vi "api_mqttSubscribe.vi"(0 "mqtt in":refnum<class "mqtt.lvclass">, 5 "subscriptionInfo":T1[](array[typedef])=[{"Topic"="a/b", "QoS"=enum."At least once"}], 9 "messageID":u16, 11 "error in (no error)":errorcluster) -> (4 "mqtt out":refnum<class "mqtt.lvclass">, 6 "success":bool, 15 "error out":errorcluster)   [LabVIEW 2020, in "mqtt.lvclass"]
uses:
  mqtt.lvclass
  mqttTypedef/mqttSubscribeCluster.ctl
  mqttTypedef/mqttQOSlevel.ctl
  mqttCmd/mqttCmdSubscribe/SubscribeMqttMsg.lvclass
  C:/Projects/Libraries/Gore SM 2020/mqtt-LabVIEW/src/class/mqtt/mqttCmd/BaseMqttMsg.lvclass
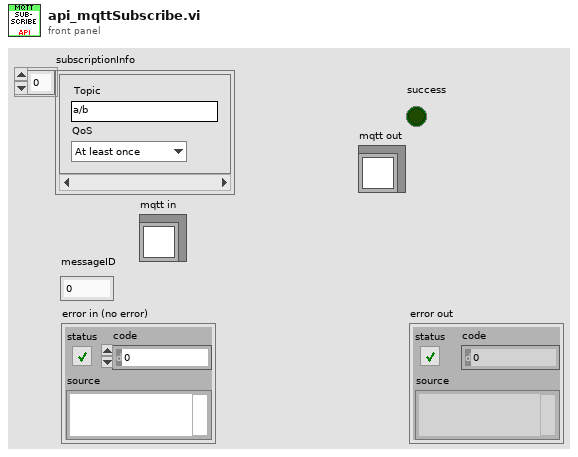
[diagram p1: front panel]
types:
  T1 = typedef "mqtt.lvclass/mqttSubscribeCluster.ctl" = cluster{"Topic":string, "QoS":T2}
  T2 = typedef "mqtt.lvclass/mqttQOSlevel.ctl" = enum8{"At most once", "At least once", "Exactly once", "Reserved"}
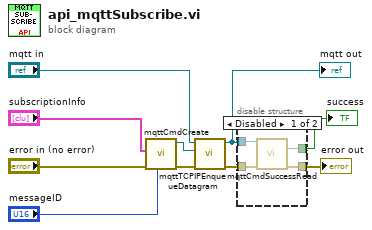
[diagram p0: block diagram]
diagram:
  n1 = call "mqttCmdCreate.vi"("messageID"="messageID", "error in (no error)"="error in (no error)", "subscriptionInfo"="subscriptionInfo") -> ("error out"=w6:errorcluster, "mqttCmdSubscribe out"=w4:refnum<class "SubscribeMqttMsg.lvclass">)  [unwired: 7 in]
  n2 = call "mqttTCPIPEnqueueDatagram.vi"("error in (no error)"=w6, "mqttCmd"=w4, "mqtt in"="mqtt in") -> ("error out"=w2:errorcluster, "mqtt out"=w1:refnum<class "mqtt.lvclass">)  [unwired: 7 in]
  "mqtt out" <- w1
  n3 = disable-structure shown="Disabled" {
    disable-tunnel: w2 -> [w14 w15]
    disable-tunnel: w1 -> [w13 _]
    disable-tunnel: [w12 w15] -> w10
    disable-tunnel: [w11 _] -> w9
    frame Disabled {
      n4 = call "mqttCmdSuccessRead.vi"("mqttBrokerCommand in"=w13, "error in (no error)"=w14) -> ("success"=w11:bool, "error out"=w12:errorcluster)  [unwired: 11 in, 1 out]
    }
    frame Enabled {
    }
  }
  "error out" <- w10
  "success" <- w9
